vi "Lense_Setup_Options.vi"() -> (1 "Focal Lengths":dbl[](array[numeric]), 3 "Lenses":string[](array[string]))   [LabVIEW 2022 SP3]
uses:
  <vilib>/Utility/error.llb/Trim Whitespace One-Sided.vi
  Globals/Constants_global.vi
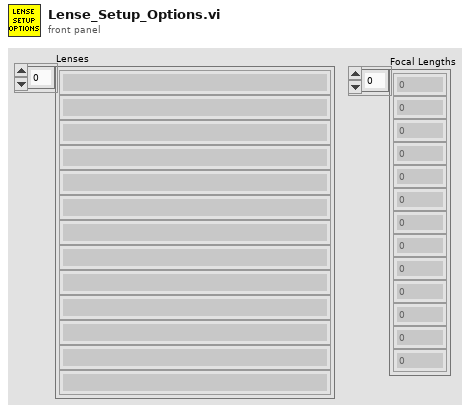
[diagram p1: front panel]
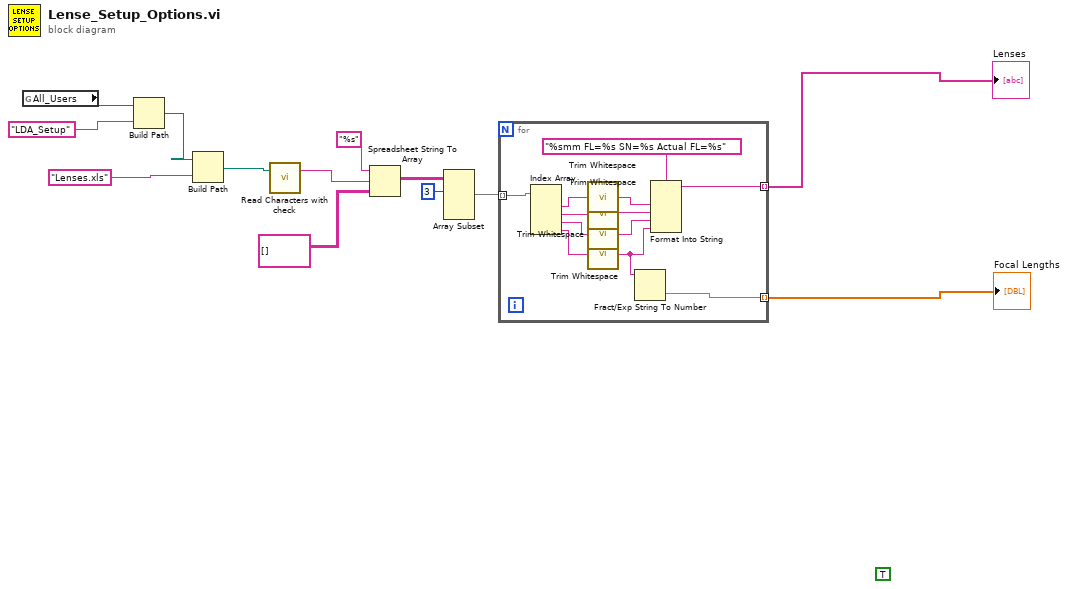
[diagram p0: block diagram]
diagram:
  (unwired) TRUE
  n1 = global read "Constants_global.vi" "All_Users"() -> (w11:path)
  n2 = Build Path(base path=w11, name or relative path="LDA_Setup") -> (appended path=w10:path)
  n3 = Build Path(base path=w10, name or relative path="Lenses.xls") -> (appended path=w2:path)
  n4 = call "Read Characters with check.vi"("file (use dialog)"=w2) -> ("Read String"=w1:string)  [unwired: 1 in, 1 out]
  n5 = Spreadsheet String To Array(format string="%s", spreadsheet string=w1, array type (2D Dbl)=string[][] []) -> (array=w7:string[][])  [unwired: 1 in]
  n6 = Array Subset(array=w7, index (row)=3 ("index")) -> (w3:string[][])  [unwired: 3 in]
  n7 = for {
    tunnel: w3 -> [w25] mode=indexing
    tunnel: [w23] -> w13 mode=indexing
    tunnel: [w14] -> w12 mode=indexing
    n8 = Index Array(array=w25) -> (element #1=w22:string, element #2=w21:string, element #3=w19:string, element #4=w18:string)  [unwired: 4 in]
    n9 = call <vilib>:"Trim Whitespace.vi"("string"=w22) -> ("trimmed string"=w15:string)  [unwired: 1 in]
    n10 = call <vilib>:"Trim Whitespace.vi"("string"=w21) -> ("trimmed string"=w20:string)  [unwired: 1 in]
    n11 = call <vilib>:"Trim Whitespace.vi"("string"=w19) -> ("trimmed string"=w17:string)  [unwired: 1 in]
    n12 = call <vilib>:"Trim Whitespace.vi"("string"=w18) -> ("trimmed string"=w16:string)  [unwired: 1 in]
    n13 = Fract/Exp String To Number(string=w16) -> (number=w14:dbl)  [unwired: 3 in, 1 out]
    n14 = Format Into String(format string="%smm FL=%s SN=%s Actual FL=%s", w15, w20, w17, w16) -> (resulting string=w23:string)  [unwired: 2 in, 1 out]
  }
  "Focal Lengths" <- w12
  "Lenses" <- w13
